vi "MW_Initialize.vi"(8 "error in (no error)":errorcluster, 11 "VISA Refnum in":refnum<visa-resource-name>) -> (0 "error out":errorcluster, 3 "VISA Refnum out":refnum<visa-resource-name>)   [LabVIEW 2016, in "Microwave Source.lvlib"]
uses:
  Microwave Source.lvlib
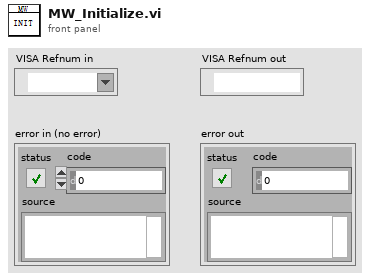
[diagram p1: front panel]
types:
  T1 = typedef "Microwave Source.lvlib/MW_ctl_DeviceType.ctl" = enum16{"R&S", "Other"}
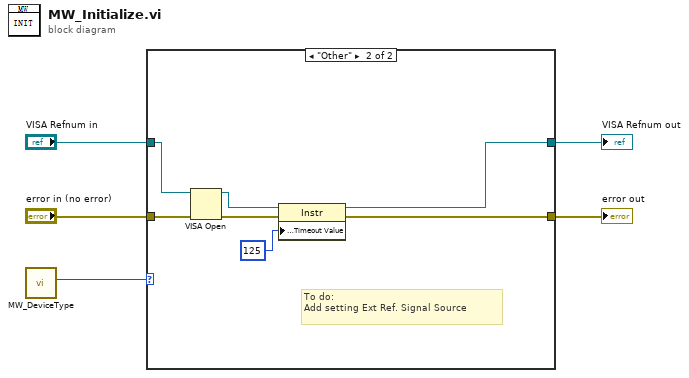
[diagram p0: block diagram]
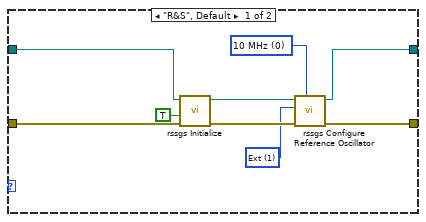
[diagram p2: hidden frame]
diagram:
  n1 = call "MW_DeviceType.vi"() -> ("DeviceType"=w1:T1)  [unwired: 11 in]
  n2 = case shown="\"Other\"" w1 {
    tunnel: "error in (no error)" -> [w14 w21]
    tunnel: "VISA Refnum in" -> [w13 w20]
    tunnel: [w8 w19] -> w3
    tunnel: [w10 w18] -> w2
    frame "R&S", Default {
      w6 = 1 items=["Int", "Ext"] ("Source (Int)")
      w7 = 0 items=["10 MHz", "100 MHz", "1000 MHz"] ("External Reference Frequency (10 MHz)")
      n3 = call <instrlib>:"rssgs Initialize.vi"("error in (no error)"=w14, "Reset Device (T)"=TRUE, "VISA resource name"=w13) -> ("error out"=w11:errorcluster, "VISA resource name out"=w9:refnum<visa-resource-name>)  [unwired: 7 in]
      n4 = call <instrlib>:"rssgs Configure Reference Oscillator.vi"("External Reference Frequency (10 MHz)"=w7, "error in (no error)"=w11, "Source (Int)"=w6, "VISA resource name"=w9) -> ("error out"=w10:errorcluster, "VISA resource name out"=w8:refnum<visa-resource-name>)  [unwired: 6 in]
    }
    frame "Other" {
      # "To do:\nAdd setting Ext Ref. Signal Source"
      n5 = VISA Open(error in (no error)=w21, VISA resource name=w20) -> (VISA resource name=w16:refnum<visa-resource-name>, error out=w17:errorcluster)  [unwired: 3 in]
      n6 = property class="Instr"(reference=w16, error in=w17, "General Settings:Timeout Value"=u32 125) -> (reference out=w19:refnum<visa-resource-name>, error out=w18:errorcluster)
    }
  }
  "VISA Refnum out" <- w3
  "error out" <- w2
